vi "Load Product and sample Metadata.vi"(8 "error in (no error)":errorcluster) -> (0 "error out":errorcluster, 3 "appended array":string[][](array[string]))   [LabVIEW 2013]
doc: "Use this template to build a standard state machine design pattern. Each state executes code and determines which state to transition to. Contrast this design pattern with the User Interface Event Handler pattern, in which code executes in response to user actions. Contrast this design pattern also with the Queued Message Handler pattern, in which each message handling code can queue zero or more new messages.\nNote: This template does not contain the most recent programming guidelines recommended by National Instruments. For a complete, project-based implementation of the Standard State Machine pattern, use the Create Project dialog box instead of this template."
uses:
  StateMachineStates 1.ctl
  <vilib>/Utility/file.llb/Read From Spreadsheet File (string).vi
panel:
  in  "Data Fields":T1
  out "Meta Data":string[][](array[string])
  in  "GO!":bool
  in  "Sample":u8=1 min=1 max=31 step=1
  in  "Model":u8=1 min=1 max=20 step=1
  # "Input the product and sample number then hit go"
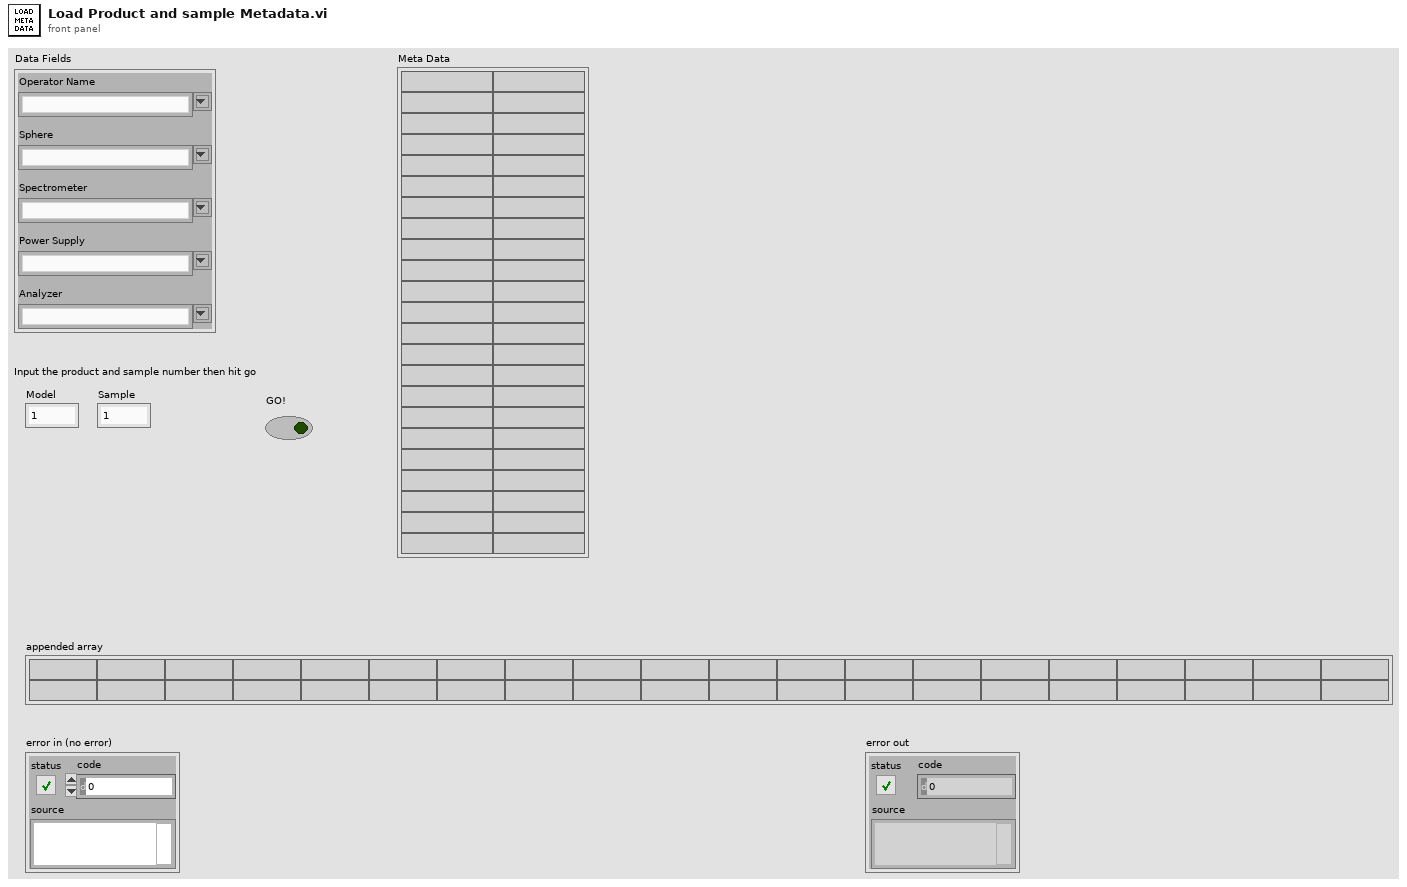
[diagram p1: front panel]
types:
  T1 = cluster{"Sphere":string, "Spectrometer":string, "Power Supply":string, "Analyzer":string, "Operator Name":string}
  T2 = typedef "StateMachineStates 1.ctl" = enum16{"Select Product and Sample", "Verify Selection", "All data entered?", "Combine metadata", "Stop"}
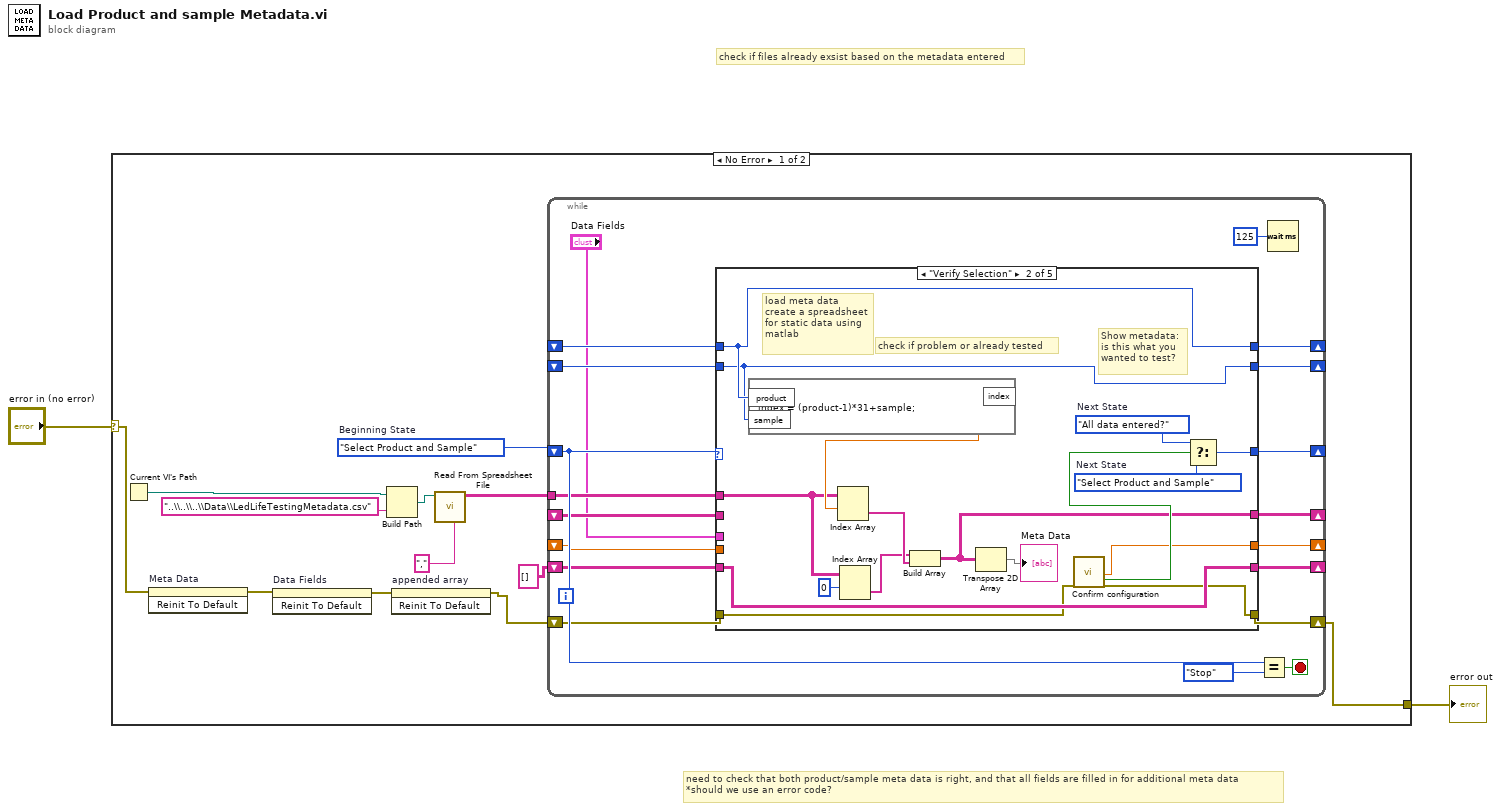
[diagram p0: block diagram]
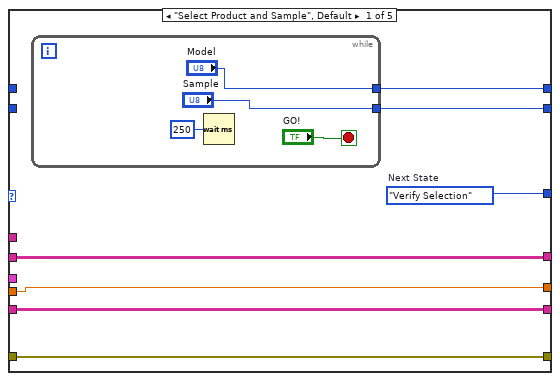
[diagram p2: hidden frame]
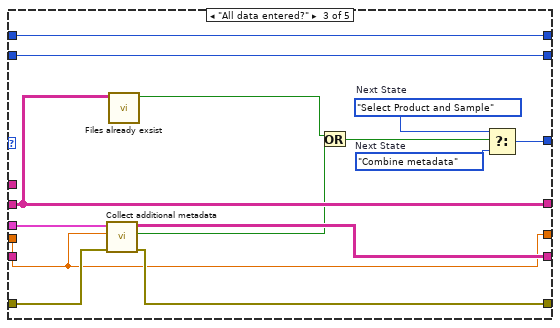
[diagram p3: hidden frame]
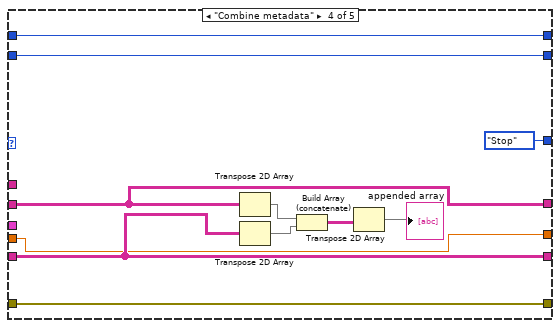
[diagram p4: hidden frame]
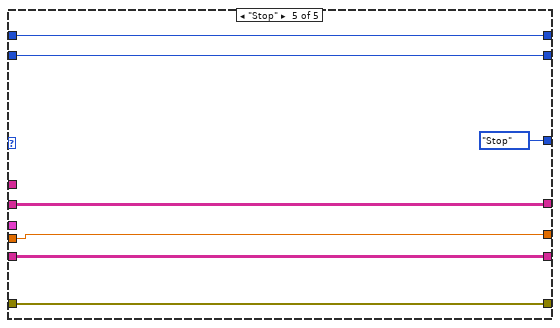
[diagram p5: hidden frame]
diagram:
  # "check if files already exsist based on the metadata entered"
  # "need to check that both product/sample meta data is right, and that all fields are filled in for additional meta data\n*should we use an error code?"
  n1 = case shown="No Error" "error in (no error)" {
    selector: "error in (no error)" -> [w8 w94]
    tunnel: [w7 w94] -> w2
    frame No Error {
      w12 = StateMachineStates_1."Select Product and Sample"  # Beginning State
      n2 = Current VI's Path() -> (path=w13:path)
      n3 = invoke on="Meta Data" class="Arr (strict)" method="Reinit To Default"(error in=w8) -> (error out=w5:errorcluster)  [unwired: 2 in, 2 out]
      n4 = invoke on="Data Fields" class="Clust (strict)" method="Reinit To Default"(error in=w5) -> (error out=w4:errorcluster)  [unwired: 2 in, 2 out]
      n5 = Build Path(base path=w13, name or relative path="..\\..\\..\\Data\\LedLifeTestingMetadata.csv") -> (appended path=w10:path)
      n6 = invoke on="appended array" class="Arr (strict)" method="Reinit To Default"(error in=w4) -> (error out=w3:errorcluster)  [unwired: 2 in, 2 out]
      n7 = call-poly <vilib>:"Read From Spreadsheet File.vi"("delimiter (\\t)"="," ("delimiter (\\t)"), "file path (dialog if empty)"=w10) -> ("all rows"=w11:string[][])  [unwired: 5 in, 4 out]
      n8 = while {
        shift-right: [w30] -> _
        shift-left: w12 -> [w31]
        shift-right: [w28] -> _
        shift-left: _ -> [w26]
        shift-right: [w27] -> _
        shift-left: _ -> [w25]
        tunnel: w11 -> [w24]
        shift-right: [w23] -> w7
        shift-left: w3 -> [w22]
        shift-right: [w18] -> _
        shift-left: string[][] [] ("appended array") -> [w21]
        shift-right: [w20] -> _
        shift-left: _ -> [w19]
        shift-right: [w16] -> _
        shift-left: _ -> [w15]
        stop <- w33 stop-if-true
        n9 = case shown="\"Verify Selection\"" w31 {
          tunnel: [w40 w61 w70 StateMachineStates_1."Stop" ("Next State") StateMachineStates_1."Stop" ("Next State")] -> w30
          tunnel: [w39 w58 w75 w86 w92] -> w28
          tunnel: [w38 w57 w74 w85 w91] -> w27
          tunnel: w26 -> [_ w58 w75 w86 w92]
          tunnel: w25 -> [_ w57 w74 w85 w91]
          tunnel: w24 -> [_ w53 _ _ _]
          tunnel: w22 -> [w37 w49 w73 w84 w90]
          tunnel: [w37 w48 w72 w84 w90] -> w23
          tunnel: [w35 w51 w68 w81 w88] -> w18
          tunnel: w21 -> [w35 w51 _ w81 w88]
          tunnel: "Data Fields" -> [_ _ w67 _ _]
          tunnel: [w36 w46 w65 w82 w89] -> w20
          tunnel: w19 -> [w36 _ w65 w82 w89]
          tunnel: [w34 w47 w66 w76 w87] -> w16
          tunnel: w15 -> [w34 _ w66 w76 w87]
          frame "Select Product and Sample", Default {
            w40 = StateMachineStates_1."Verify Selection"  # Next State
            n10 = while {
              tunnel: ["Model"] -> w39
              tunnel: ["Sample"] -> w38
              stop <- "GO!" stop-if-true
              n11 = Wait (ms)(milliseconds to wait=u32 250) -> ()  [unwired: 1 out]
            }
          }
          frame "Verify Selection" {
            w59 = StateMachineStates_1."Select Product and Sample"  # Next State
            w60 = StateMachineStates_1."All data entered?"  # Next State
            # "Show metadata:\nis this what you \nwanted to test?"
            # "check if problem or already tested"
            # "load meta data\ncreate a spreadsheet\nfor static data using\nmatlab"
            n12 = formula code="index = (product-1)*31+sample;"("product"=w58, "sample"=w57) -> ("index"=w56:dbl)
            n13 = Index Array(array=w53, index (row)=w56) -> (element=w55:string[])  [unwired: 1 in]
            n14 = Index Array(array=w53, index (row)=0) -> (element=w52:string[])  [unwired: 1 in]
            n15 = Build Array(w52, w55) -> (w46:string[][])
            n16 = Transpose 2D Array(2D array=w46) -> (transposed array=→"Meta Data":string[][])
            n17 = call "Confirm configuration"("error in (no error)"=w49) -> ("Run time hours"=w47:dbl, "OK"=w50:bool, "error out"=w48:errorcluster)  [unwired: 16 in]
            n18 = Select(t=w60, s=w50, f=w59) -> (s? t:f=w61:T2)
          }
          frame "All data entered?" {
            w69 = StateMachineStates_1."Combine metadata"  # Next State
            w71 = StateMachineStates_1."Select Product and Sample"  # Next State
            n19 = call "Collect additional metadata.vi"("error in (no error)"=w73, "hours"=w66, "Data Fields"=w67) -> ("error out"=w72:errorcluster, "Error"=w64:bool, "appended array"=w68:string[][])  [unwired: 6 in]
            n20 = call "Files already exsist.vi"("Array"=w65) -> ("Files already exsist"=w62:bool)  [unwired: 10 in]
            n21 = Or(x=w62, y=w64) -> (x .or. y?=w63:bool)
            n22 = Select(t=w71, s=w63, f=w69) -> (s? t:f=w70:T2)
          }
          frame "Combine metadata" {
            n23 = Transpose 2D Array(2D array=w82) -> (transposed array=w80:string[][])
            n24 = Transpose 2D Array(2D array=w81) -> (transposed array=w79:string[][])
            n25 = Build Array (concatenate)(w80, w79) -> (w78:string[][])
            n26 = Transpose 2D Array(2D array=w78) -> (transposed array=→"appended array":string[][])
          }
          frame "Stop" {
          }
        }
        n27 = Equal?(x=w31, y=StateMachineStates_1."Stop" ("States")) -> (x = y?=w33:bool)
        n28 = Wait (ms)(milliseconds to wait=u32 125) -> ()  [unwired: 1 out]
      }
    }
    frame Error {
    }
  }
  "error out" <- w2
